vi "Main Tree _ Add VCH Tag.vi"(8 "error in":errorcluster caption="错误输入", 11 "Ref.Tree Ref":refnum<vi>) -> (0 "error out":errorcluster caption="错误输出")   [LabVIEW 2016]
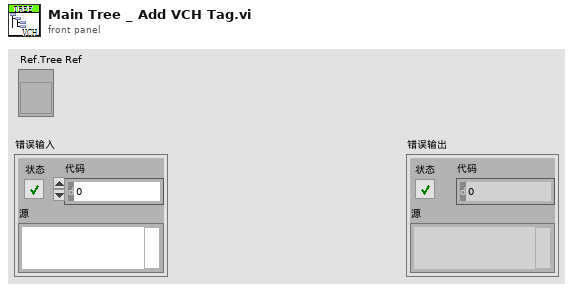
[diagram p1: front panel]
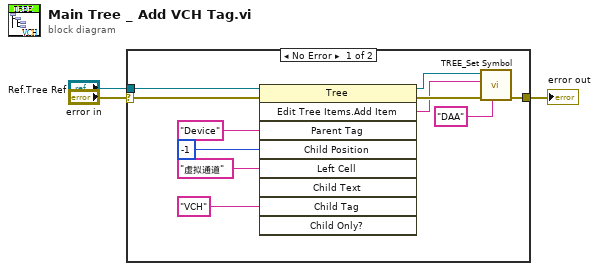
[diagram p0: block diagram]
diagram:
  n1 = case shown="No Error" "error in" {
    selector: "error in" -> [w13 w15]
    tunnel: [w11 w15] -> w2
    tunnel: "Ref.Tree Ref" -> [w14 _]
    frame No Error {
      n2 = invoke class="Tree" method="Edit Tree Items.Add Item"(reference=w14, error in=w13, "Parent Tag"="Device", "Child Position"=-1 ("子项位置"), "Left Cell"="虚拟通道", "Child Tag"="VCH") -> (reference out=w10:refnum<vi>, error out=w9:errorcluster, "Edit Tree Items:Add Item"=w8:string)  [unwired: 3 in, 6 out]
      n3 = call "TREE_Set Symbol.vi"("PicName"="DAA", "error in"=w9, "Tag"=w8, "Tree Ref"=w10) -> ("error out"=w11:errorcluster)  [unwired: 6 in, 1 out]
    }
    frame Error {
    }
  }
  "error out" <- w2
